vi "Launch Logging Manager.vi"(8 "error in (no error)":errorcluster, 9 "Logging Root":path, 10 "VolatusAPI":refnum<class "VolatusAPI.lvclass">, 11 "Config Element":refnum<class "Config Element.lvclass">) -> (0 "error out":errorcluster, 2 "LoggingAPI":refnum<class "LoggingAPI.lvclass">)   [LabVIEW 2020, in "VolatusDataLogger.lvlib" / "LoggingManager.lvclass"]
uses:
  LoggingManager.lvclass
  LoggingAPI/LoggingAPI.lvclass
  Volatus/VolatusAPI/VolatusAPI.lvclass
  C:/dev/lv20CE/relink/lv-volatus/Volatus/Task/Task.lvclass
  LoggingManager.lvclass/LoggingManager.ctl
  C:/Program Files (x86)/National Instruments/LabVIEW 2020/vi.lib/ActorFramework/Actor/Actor.lvclass
  C:/dev/lv20CE/relink/lv-volatus/Volatus/TaskStateHandler/TaskStateHandler.lvclass
  C:/dev/lv20CE/relink/lv-volatus/Volatus/VectoMessageHandler/VectoMessageHandler.lvclass
  C:/dev/lv20CE/relink/lv-volatus/VolatusDataLogger/LoggingManager/LoggingManager.lvclass
  C:/dev/lv20CE/relink/lv-volatus/Volatus/API Provider/API Provider.lvclass
  C:/dev/lv20CE/relink/lv-volatus/VolatusDataLogger/LoggingHandler/LoggingHandler.lvclass
  Volatus/Task/Task.lvclass
  lv-cdm/CDM-Config/Config Element/Config Element.lvclass
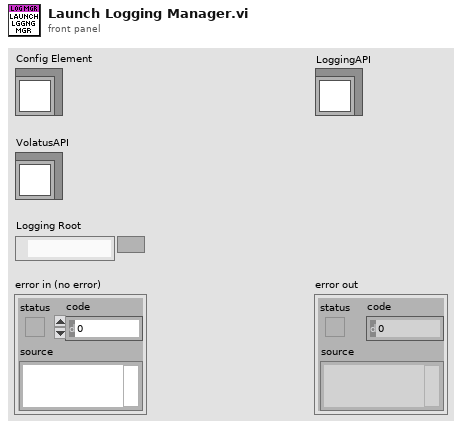
[diagram p1: front panel]
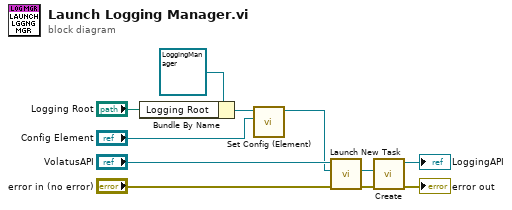
[diagram p0: block diagram]
diagram:
  n1 = Bundle By Name(cluster=refnum<class "LoggingManager.lvclass"> refnum ("VolatusDataLogger:LoggingManager"), "Logging Root"="Logging Root") -> (w4:refnum<class "LoggingManager.lvclass">)
  n2 = call "Set Config (Element).vi"("Config Element"="Config Element", "Task in"=w4) -> ("Task out"=w2:refnum<class "LoggingManager.lvclass">)  [unwired: 8 in, 1 out]
  n3 = call "Launch New Task.vi"("error in (no error)"="error in (no error)", "Task"=w2, "VolatusAPI in"="VolatusAPI") -> ("error out"=w8:errorcluster, "EnQr"=w9:refnum<class "Message Enqueuer.lvclass">)  [unwired: 6 in, 1 out]
  n4 = call "Create.vi"("error in (no error)"=w8, "EnQr"=w9) -> ("error out"=→"error out":errorcluster, "LoggingAPI out"=→"LoggingAPI":refnum<class "LoggingAPI.lvclass">)  [unwired: 8 in]
